vi "Results from Cam 2.vi"(7 "Image Nr.":i32, 8 "error in (no error)":errorcluster, 9 "Parameters":refnum<class "Analyze Parameter Base.lvclass">[](array[class]), 10 "Results":refnum<class "Analyze Results Base.lvclass">[](array[class]), 11 "HIJ Multiple Cams App Demo in":refnum<class "HIJ 4 Alignment Cams App.lvclass">) -> (0 "error out":errorcluster, 3 "HIJ Multiple Cams App Demo out":refnum<class "HIJ 4 Alignment Cams App.lvclass">)   [LabVIEW 2014]
uses:
  HIJ 4 Alignment Cams App.lvclass
  Analyze/Results and Overlays/Results Base/Analyze Results Base.lvclass
  Analyze/Analyze Parameter/Analyze Parameter Base/Analyze Parameter Base.lvclass
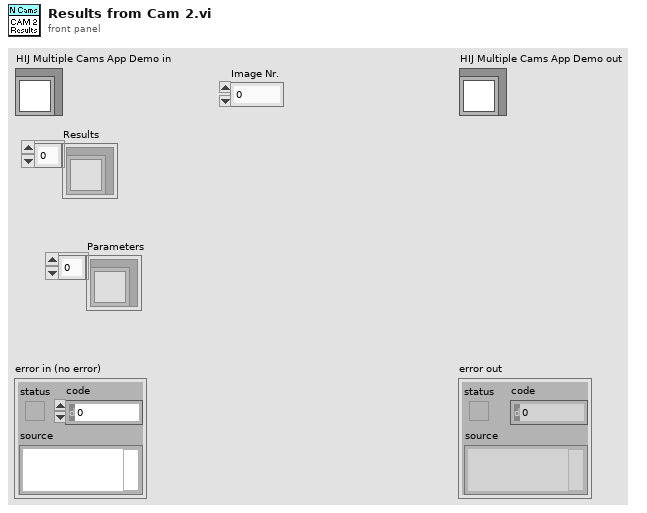
[diagram p1: front panel]
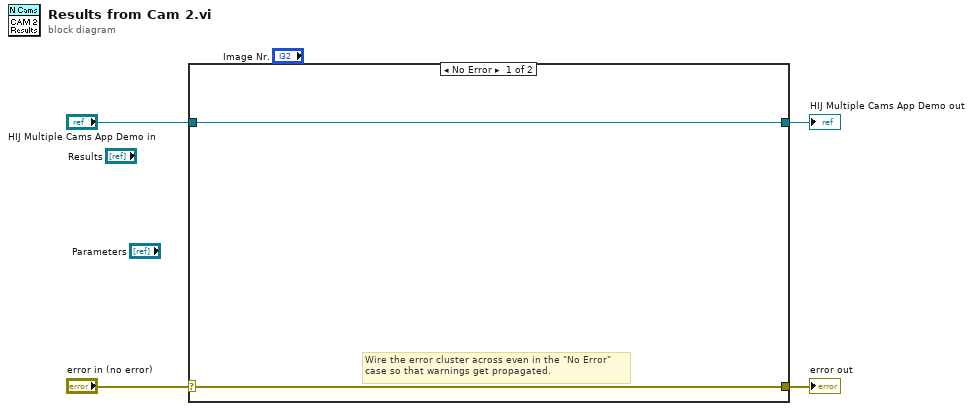
[diagram p0: block diagram]
diagram:
  n1 = case shown="No Error" "error in (no error)" {
    selector: "error in (no error)" -> [w5 w8]
    tunnel: [w5 w8] -> w3
    tunnel: [w6 w7] -> w1
    tunnel: "HIJ Multiple Cams App Demo in" -> [w6 w7]
    frame No Error {
      # "Wire the error cluster across even in the \"No Error\"\ncase so that warnings get propagated."
    }
    frame Error {
    }
  }
  "error out" <- w3
  "HIJ Multiple Cams App Demo out" <- w1
